vi "HtmlPrepareGithub.vi"() -> ()   [LabVIEW 2024]
panel:
  in  "Remove LibaryName":string="OpenLvVision_Image.lvlib:Management.lvlib:"
  out "error out":errorcluster
  in  "Images":string[][](array[string])=[["cbool.png", "https://github.com/user-attachments/assets/12205308-27f0-4cd2-936f-db5a8b190330"], ["cenum.png", "https://github.com/user-attachments/assets/05d9c66f-1eef-4069-a6ca-453150029222"], ["cerrcodeclst.png", "https://github.com/user-attachments/assets/29c25b91-7c92-4aa1-8c7e-b9e61b1e84e2"], ["ci32.png", "https://github.com/user-attachments/assets/3d2c108b-8fd9-4834-bfb4-9142a681c912"], ["cstr.png", "https://github.com/user-attachments/assets/67ac2589-cb7f-482d-ac4d-5c871636be71"]]
  # "Image Name"
  # "URL"
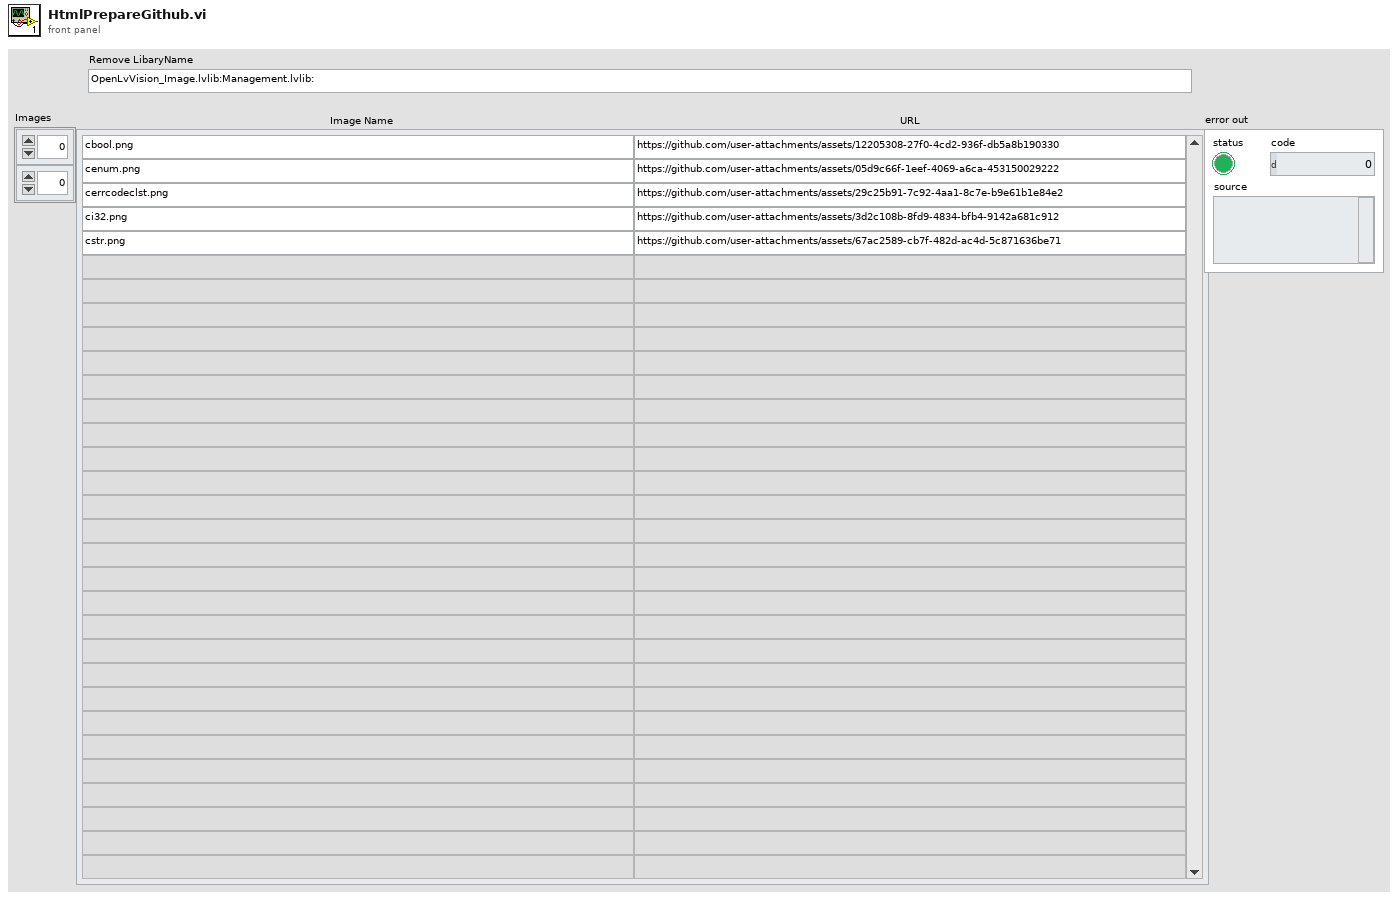
[diagram p1: front panel]
types:
  T1 = enum16{"open", "replace", "create", "open or create", "replace or create", "replace or create with confirmation"}
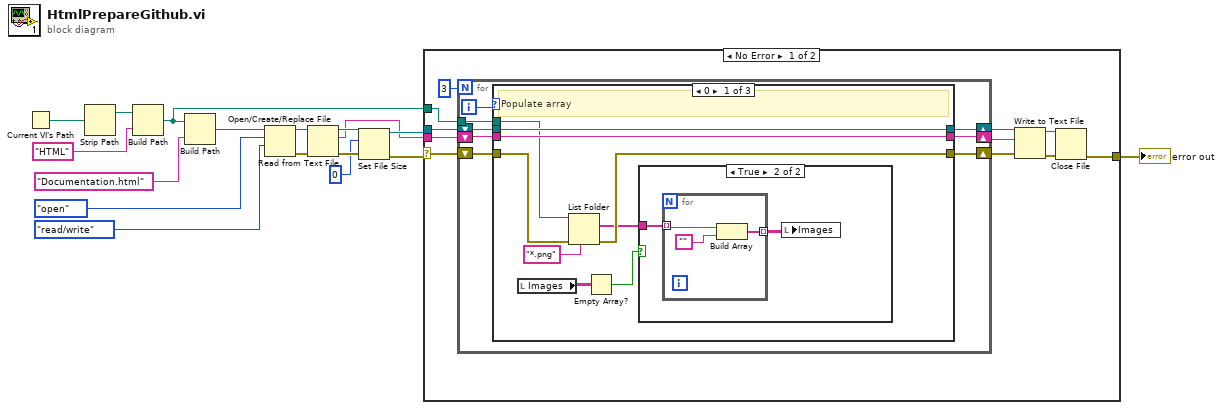
[diagram p0: block diagram]
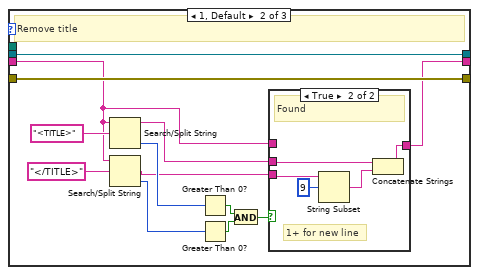
[diagram p3: hidden frame]
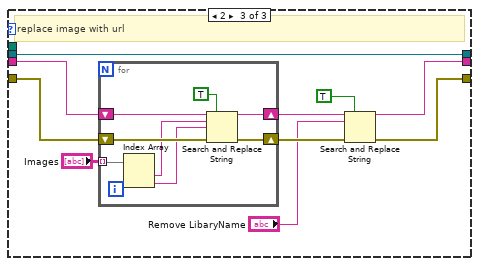
[diagram p5: hidden frame]
diagram:
  n1 = Current VI's Path() -> (path=w15:path)
  n2 = Strip Path(path=w15) -> (stripped path=w14:path)  [unwired: 1 out]
  n3 = Build Path(base path=w14, name or relative path="HTML") -> (appended path=w1:path)
  n4 = Build Path(base path=w1, name or relative path="Documentation.html") -> (appended path=w10:path)
  n5 = Open/Create/Replace File(file path (use dialog)=w10, operation (0:open)=T1."open", access (0:read/write)=enum16{"read/write", "read-only", "write-only"}."read/write") -> (refnum out=w11:refnum<file>, error out=w12:errorcluster)  [unwired: 3 in, 1 out]
  n6 = Read from Text File(file (use dialog)=w11, error in=w12) -> (refnum out=w6:refnum<file>, text=w2:string, error out=w7:errorcluster)  [unwired: 2 in, 1 out]
  n7 = Set File Size(4:w7, 6:i64 0 ("size (in bytes)"), 7:w6) -> (0:w4:errorcluster, 3:w5:refnum<file>)
  n8 = case shown="No Error" w4 {
    selector: w4 -> [w25 w88]
    tunnel: w2 -> [w28 _]
    tunnel: w5 -> [w26 _]
    tunnel: [w20 w88] -> w13
    tunnel: w1 -> [w18 _]
    frame No Error {
      n9 = for {
        N: 3 -> [_]
        shift-right: [w30] -> w23
        shift-left: w25 -> [w31]
        shift-right: [w34] -> w19
        shift-left: w26 -> [w35]
        shift-right: [w32] -> w24
        shift-left: w28 -> [w33]
        tunnel: w18 -> [w29]
        i -> [w36]
        # "remove title"
        n10 = case shown="0" w36 {
          tunnel: w35 -> [w45 w63 w79]
          tunnel: [w45 w63 w79] -> w34
          tunnel: w33 -> [w44 w52 w77]
          tunnel: [w44 w51 w73] -> w32
          tunnel: w31 -> [w42 w60 w76]
          tunnel: [w40 w60 w72] -> w30
          tunnel: w29 -> [w43 _ _]
          frame 0 {
            # "Populate array"
            n11 = local read "Images"() -> (w38:string[][])
            n12 = List Folder(path=w43, pattern="*.png", error in=w42) -> (filenames=w39:string[], error out=w40:errorcluster)  [unwired: 1 in, 2 out]
            n13 = Empty Array?(array=w38) -> (empty?=w37:bool)
            n14 = case shown="True" w37 {
              tunnel: w39 -> [_ w47]
              frame False {
              }
              frame True {
                n15 = for {
                  tunnel: w47 -> [w50] mode=indexing
                  tunnel: [w48] -> w46 mode=indexing
                  n16 = Build Array(w50, "") -> (w48:string[])
                }
                n17 = local write "Images"(w46) -> ()
              }
            }
          }
          frame 1, Default {
            # "Remove title"
            n18 = Search/Split String(string=w52, search string/char (-)="<TITLE>") -> (substring before match=w54:string, offset of match=w56:i32)  [unwired: 1 in, 1 out]
            n19 = Search/Split String(string=w52, search string/char (-)="</TITLE>") -> (match + rest of string=w53:string, offset of match=w57:i32)  [unwired: 1 in, 1 out]
            n20 = Greater Than 0?(x=w56) -> (x > 0?=w62:bool)
            n21 = Greater Than 0?(x=w57) -> (x > 0?=w61:bool)
            n22 = And(x=w62, y=w61) -> (x .and. y?=w55:bool)
            n23 = case shown="True" w55 {
              tunnel: w54 -> [_ w67]
              tunnel: w53 -> [_ w69]
              tunnel: w52 -> [w64 _]
              tunnel: [w64 w65] -> w51
              frame False {
                # "not found"
              }
              frame True {
                # "1+ for new line"
                # "Found"
                n24 = String Subset(string=w69, offset (0)=9) -> (substring=w66:string)  [unwired: 1 in]
                n25 = Concatenate Strings(w67, w66) -> (w65:string)
              }
            }
          }
          frame 2 {
            # "replace image with url"
            n26 = for {
              tunnel: "Images" -> [w87] mode=indexing
              shift-right: [w85] -> w74
              shift-left: w77 -> [w86]
              shift-right: [w82] -> w75
              shift-left: w76 -> [w83]
              # "Build html search"
              n27 = Index Array(array=w87) -> (element #1=w81:string, element #2=w80:string)  [unwired: 2 in]
              n28 = Search and Replace String(replace all?=TRUE, input string=w86, search string=w81, replace string=w80, error in=w83) -> (result string=w85:string, error out=w82:errorcluster)  [unwired: 3 in, 2 out]
            }
            n29 = Search and Replace String(replace all?=TRUE, input string=w74, search string="Remove LibaryName", error in=w75) -> (result string=w73:string, error out=w72:errorcluster)  [unwired: 4 in, 2 out]
          }
        }
      }
      n30 = Write to Text File(file (use dialog)=w19, text=w24, error in=w23) -> (refnum out=w21:refnum<file>, error out=w22:errorcluster)  [unwired: 1 in, 1 out]
      n31 = Close File(refnum=w21, error in=w22) -> (error out=w20:errorcluster)  [unwired: 1 out]
    }
    frame Error {
    }
  }
  "error out" <- w13
